vi "Read-Save Bands.vi"(6 "Task":enum16{"Save", "Read", "List"}(ring)=enum."List", 9 "Name":string="favorites.txt", 11 "Frequencies":dbl[](array[numeric])=[440.0]) -> (0 "file names":string[](array[string]), 1 "String":string, 2 "Long names":string[](array[string]), 3 "Frequencies":dbl[](array[numeric])=[440.0])   [LabVIEW 2022 SP3]
uses:
  <vilib>/Utility/error.llb/Trim Whitespace One-Sided.vi
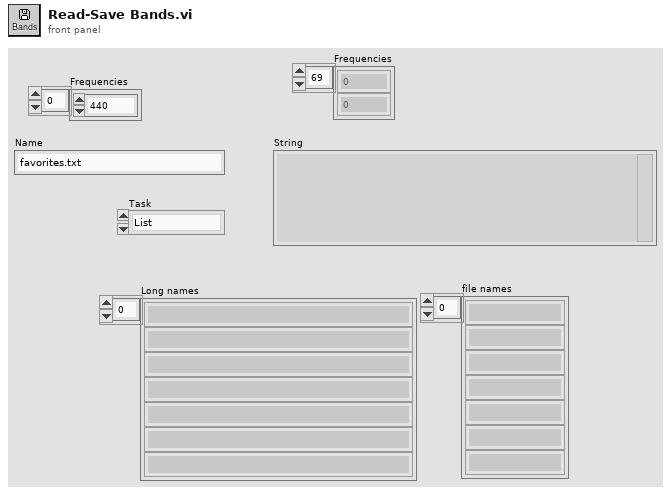
[diagram p1: front panel]
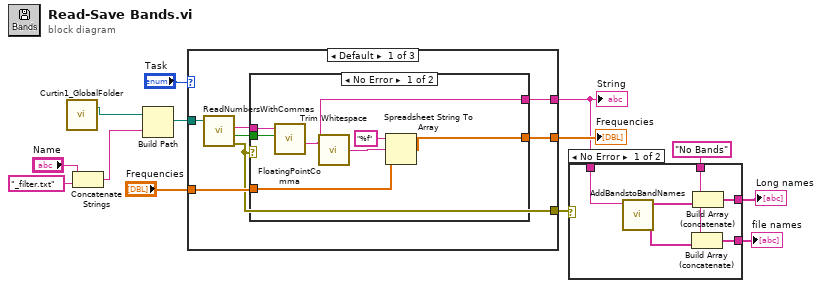
[diagram p0: block diagram]
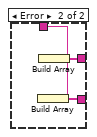
[diagram p2: hidden frame]
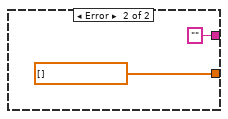
[diagram p3: hidden frame]
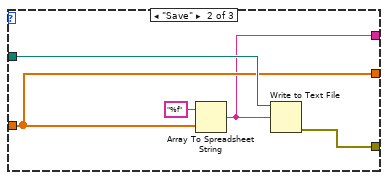
[diagram p4: hidden frame]
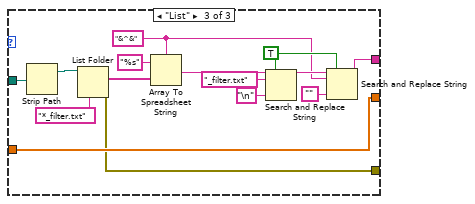
[diagram p5: hidden frame]
diagram:
  n1 = call "Curtin1_GlobalFolder.vi"() -> ("LabVIEW Data Path"=w2:path)  [unwired: 1 in, 1 out]
  n2 = Concatenate Strings("Name", "_filter.txt" ("string")) -> (w7:string)
  n3 = Build Path(base path=w2, name or relative path=w7) -> (appended path=w12:path)
  n4 = case shown="Default" "Task" {
    tunnel: "Frequencies" -> [w19 w32 w49]
    tunnel: w12 -> [w17 w34 w48]
    tunnel: [w16 w33 w42] -> w3
    tunnel: [w20 w32 w49] -> w10
    tunnel: [w18 w30 w36] -> w5
    frame Default {
      n5 = call "ReadNumbersWithCommas.vi"("file (use dialog)"=w17) -> ("error out"=w16:errorcluster, "comma?"=w14:bool, "text"=w15:string)  [unwired: 7 in, 1 out]
      n6 = case shown="No Error" w16 {
        tunnel: [w25 dbl[] [] ("DataPath")] -> w20
        tunnel: w15 -> [w23 _]
        tunnel: w19 -> [w27 _]
        tunnel: [w21 ""] -> w18
        tunnel: w14 -> [w22 _]
        frame No Error {
          n7 = call "FloatingPointComma.vi"("Comma?"=w22, "String In"=w23) -> ("fixed"=w21:string)  [unwired: 8 in, 1 out]
          n8 = call <vilib>:"Trim Whitespace.vi"("string"=w21) -> ("trimmed string"=w24:string)  [unwired: 1 in]
          n9 = Spreadsheet String To Array(format string="%f", spreadsheet string=w24, array type (2D Dbl)=w27) -> (array=w25:dbl[])  [unwired: 1 in]
        }
        frame Error {
        }
      }
    }
    frame "Save" {
      n10 = Array To Spreadsheet String(array=w32, 3:"%f" ("format string")) -> (spreadsheet string=w30:string)  [unwired: 1 in]
      n11 = Write to Text File(file (use dialog)=w34, text=w30) -> (error out=w33:errorcluster)  [unwired: 2 in, 2 out]
    }
    frame "List" {
      w35 = "&^&" ("delimiter (Tab)")
      w38 = TRUE ("replace all? (F)")
      n12 = Strip Path(path=w48) -> (stripped path=w47:path)  [unwired: 1 out]
      n13 = List Folder(path=w47, pattern="*_filter.txt") -> (filenames=w45:string[], error out=w42:errorcluster)  [unwired: 2 in, 2 out]
      n14 = Array To Spreadsheet String(delimiter (Tab)=w35, array=w45, 3:"%s" ("format string")) -> (spreadsheet string=w37:string)
      n15 = Search and Replace String(replace all?=w38, input string=w37, search string="_filter.txt", replace string="\n" ("replace string (\"\")")) -> (result string=w39:string)  [unwired: 4 in, 3 out]
      n16 = Search and Replace String(replace all?=w38, input string=w39, search string=w35, replace string="" ("replace string (\"\")")) -> (result string=w36:string)  [unwired: 4 in, 3 out]
    }
  }
  "Frequencies" <- w10
  "String" <- w5
  n17 = case shown="No Error" w3 {
    tunnel: "No Bands" ("String") -> [w51 w56]
    tunnel: w5 -> [w54 _]
    tunnel: [w53 w58] -> w4
    tunnel: [w50 w57] -> w1
    frame No Error {
      n18 = call "AddBandstoBandNames.vi"("filter name"=w54) -> ("File Name"=w52:string[], "Extended Name"=w55:string[])  [unwired: 9 in]
      n19 = Build Array (concatenate)(w51, w52) -> (w50:string[])
      n20 = Build Array (concatenate)(w51, w55) -> (w53:string[])
    }
    frame Error {
      n21 = Build Array(w56) -> (w57:string[])
      n22 = Build Array(w56) -> (w58:string[])
    }
  }
  "Long names" <- w4
  "file names" <- w1
